vi "DetermineCommand.vi"(9 "cmd":string="import os\nos.system('')", 11 "Console":string) -> (1 "python?":bool=TRUE, 3 "cmd out":string)   [LabVIEW 2022 SP3]
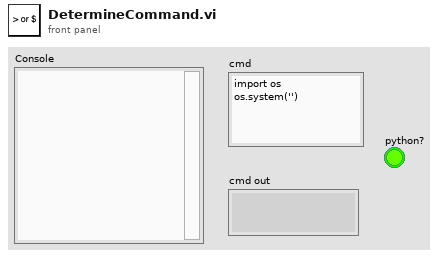
[diagram p1: front panel]
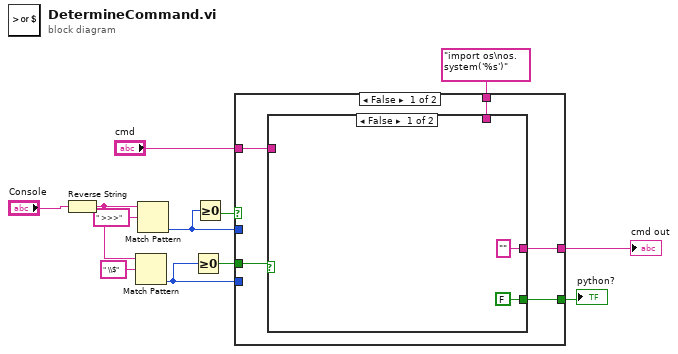
[diagram p0: block diagram]
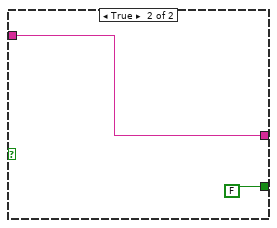
[diagram p2: hidden frame]
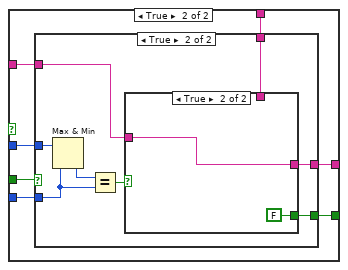
[diagram p3: hidden frame]
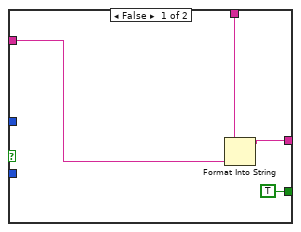
[diagram p4: hidden frame]
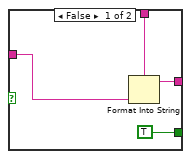
[diagram p5: hidden frame]
diagram:
  n1 = Reverse String(1:"Console") -> (0:w11:string)
  n2 = Match Pattern(string=w11, regular expression=" \\$") -> (offset past match=w5:i32)  [unwired: 1 in, 3 out]
  n3 = Match Pattern(string=w11, regular expression=" >>>") -> (offset past match=w6:i32)  [unwired: 1 in, 3 out]
  n4 = Greater Or Equal To 0?(x=w5) -> (x >= 0?=w3:bool)
  n5 = Greater Or Equal To 0?(x=w6) -> (x >= 0?=w4:bool)
  n6 = case shown="False" w4 {
    tunnel: [w14 w28] -> w12
    tunnel: "cmd" -> [w16 w27]
    tunnel: w6 -> [_ w26]
    tunnel: w5 -> [_ w25]
    tunnel: w3 -> [w17 w24]
    tunnel: "import os\nos.system('%s')" ("python 2") -> [w15 w23]
    tunnel: [w13 w22] -> w1
    frame False {
      n7 = case shown="False" w17 {
        tunnel: w16 -> [_ w21]
        tunnel: w15 -> [_ _]
        tunnel: ["" w21] -> w14
        tunnel: [FALSE FALSE] -> w13
        frame False {
        }
        frame True {
        }
      }
    }
    frame True {
      n8 = case shown="True" w24 {
        tunnel: [w30 w40] -> w28
        tunnel: w27 -> [w32 w37]
        tunnel: w26 -> [_ w36]
        tunnel: w25 -> [_ w35]
        tunnel: w23 -> [w31 w34]
        tunnel: [TRUE w33] -> w22
        frame False {
          n9 = Format Into String(format string=w31, w32) -> (resulting string=w30:string)  [unwired: 2 in, 1 out]
        }
        frame True {
          n10 = Max & Min(x=w36, y=w35) -> (min(x,y)=w39:i32)  [unwired: 1 out]
          n11 = Equal?(x=w39, y=w35) -> (x = y?=w38:bool)
          n12 = case shown="True" w38 {
            tunnel: [w43 w46] -> w40
            tunnel: w37 -> [w44 w46]
            tunnel: w34 -> [w42 _]
            tunnel: [TRUE FALSE] -> w33
            frame False {
              n13 = Format Into String(format string=w42, w44) -> (resulting string=w43:string)  [unwired: 2 in, 1 out]
            }
            frame True {
            }
          }
        }
      }
    }
  }
  "cmd out" <- w12
  "python?" <- w1
